vi "AO and DO Engine.vi"(0 "Unique Notifier Name":string="Not a Name", 11 "AO Channel":string[](array[string])) -> ()   [LabVIEW 2016]
uses:
  External Power Control Type Defs/External Power Notifier Type.ctl
  External Power Control Type Defs/External Power Actions.ctl
  <vilib>/DAQmx/write.llb/DAQmx Write (Digital Bool 1Line 1Point).vi
  <vilib>/DAQmx/write.llb/DAQmx Write (Analog DBL 1Chan 1Samp).vi
  <vilib>/DAQmx/create/channels.llb/DAQmx Create Channel (DO-Digital Output).vi
  <vilib>/DAQmx/miscellaneous.llb/DAQmx Fill In Error Info.vi
  <vilib>/DAQmx/create/channels.llb/DAQmx Create Channel (AO-Voltage-Basic).vi
panel:
  in  "Power (%)":dbl
  in  "Quit":bool
  in  "Line On Off":bool
  # "Array Elements must be:\n\n1) AO Channel (e.g. Dev1/ao3)\n2) DO Channel (e.g. Dev1/port0/line16)"
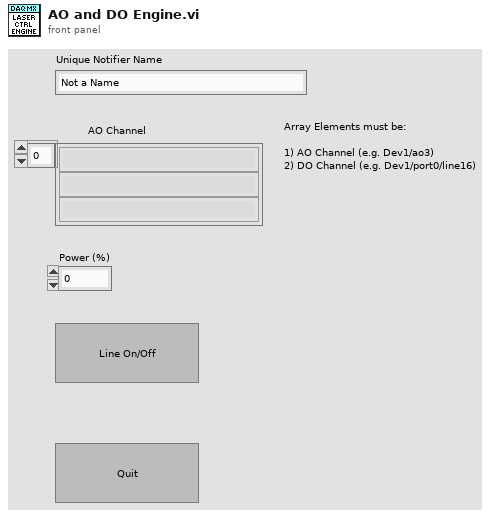
[diagram p1: front panel]
types:
  T1 = typedef "External Power Notifier Type.ctl" = cluster{"Actions":T2, "Wavelength":string, "Line On/Off":bool, "Power (%)":dbl, "Control Parameters":variant, "Cmd Done?":bool}
  T2 = typedef "External Power Actions.ctl" = enum16{"Line On/Off", "Set Power", "Set Ctrl Parameters", "Quit"}
  T3 = enum32{"Invalid", "Standard", "Closed", "Hidden", "Minimized", "Maximized"}
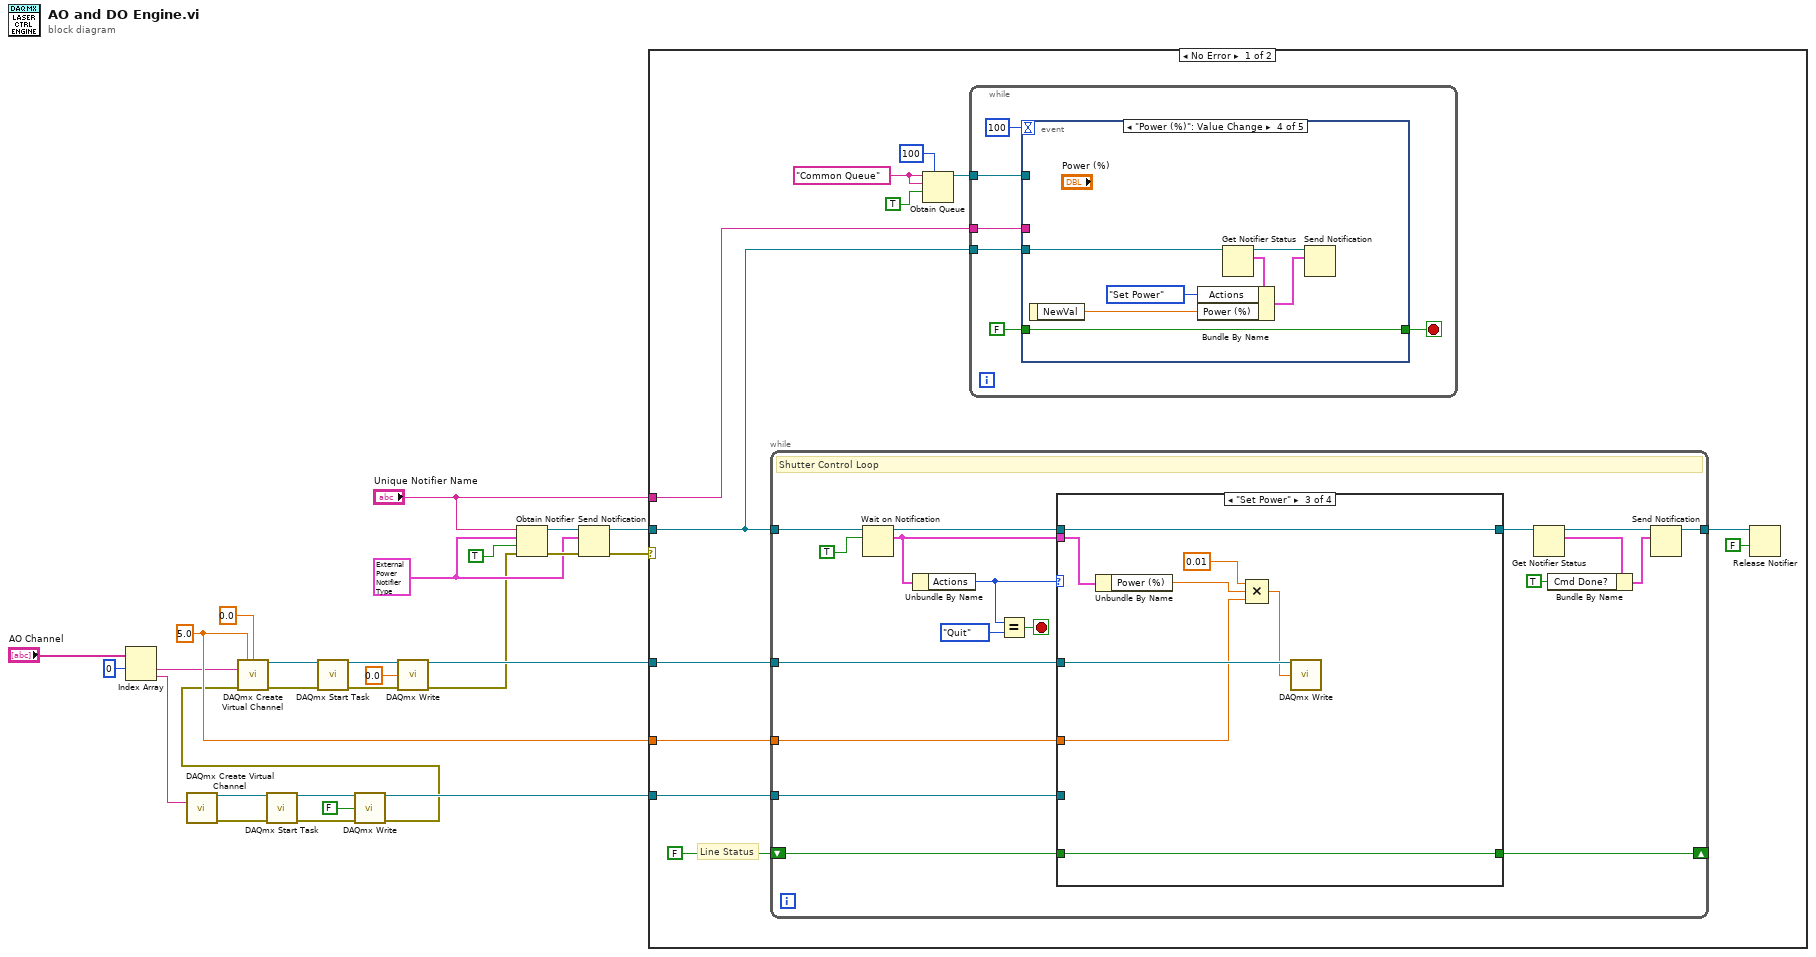
[diagram p0: block diagram]
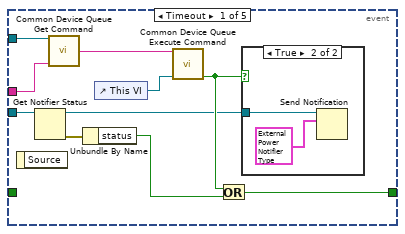
[diagram p2: hidden frame]
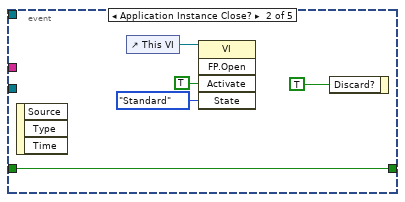
[diagram p4: hidden frame]
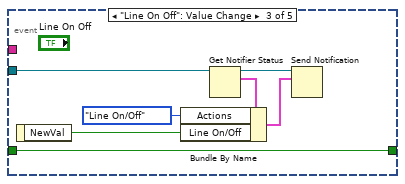
[diagram p5: hidden frame]
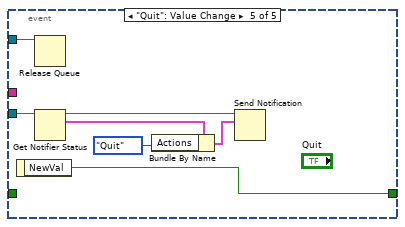
[diagram p6: hidden frame]
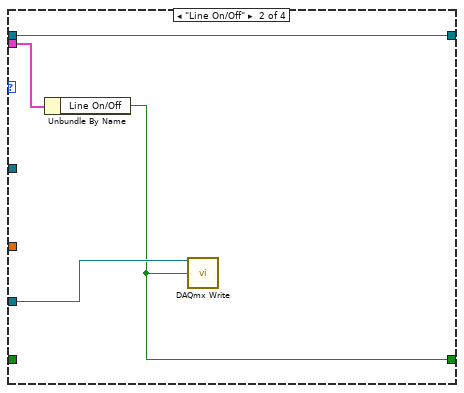
[diagram p8: hidden frame]
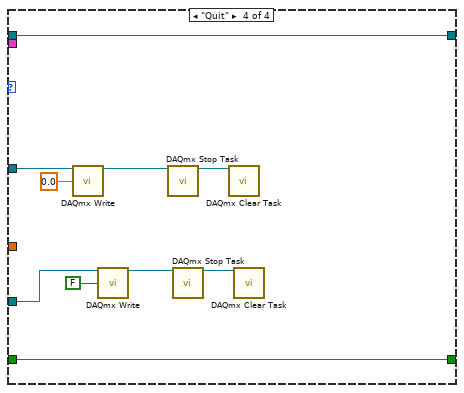
[diagram p9: hidden frame]
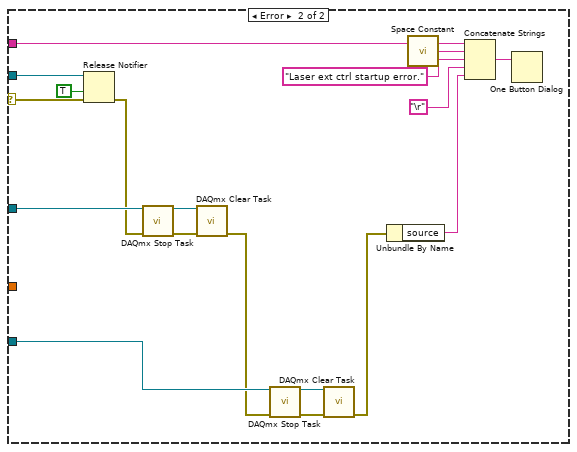
[diagram p10: hidden frame]
diagram:
  w18 = 5.0 ("maximum value")
  w23 = T1 {"Actions"=enum."Set Power", "Wavelength"="", "Line On/Off"=FALSE, "Power (%)"=0.0, "Control Parameters"=variant, "Cmd Done?"=FALSE} ("External Ctrl")
  n1 = Index Array(array="AO Channel", index #1=0 ("index")) -> (element #1=w9:string, element #2=w1:string)  [unwired: 1 in]
  n2 = call-poly <vilib>:"DAQmx Create Virtual Channel.vi"("lines"=w1) -> ("task out"=w7:refnum<k21>, "error out"=w8:errorcluster)  [unwired: 13 in]
  n3 = call <vilib>:"DAQmx Start Task.vi"("task/channels in"=w7, "error in"=w8) -> ("task out"=w6:refnum<k21>, "error out"=w4:errorcluster)  [unwired: 12 out]
  n4 = call-poly <vilib>:"DAQmx Write.vi"("task/channels in"=w6, "data"=FALSE, "error in"=w4) -> ("task out"=w3:refnum<k21>, "error out"=w2:errorcluster)  [unwired: 10 in, 1 out]
  n5 = call-poly <vilib>:"DAQmx Create Virtual Channel.vi"("maximum value"=w18, "minimum value"=0.0, "physical channels"=w9, "error in"=w2) -> ("task out"=w14:refnum<k21>, "error out"=w13:errorcluster)  [unwired: 10 in]
  n6 = call <vilib>:"DAQmx Start Task.vi"("task/channels in"=w14, "error in"=w13) -> ("task out"=w12:refnum<k21>, "error out"=w11:errorcluster)  [unwired: 12 out]
  n7 = call-poly <vilib>:"DAQmx Write.vi"("task/channels in"=w12, "data"=0.0, "error in"=w11) -> ("task out"=w16:refnum<k21>, "error out"=w10:errorcluster)  [unwired: 10 in, 1 out]
  n8 = Obtain Notifier(name (unnamed)="Unique Notifier Name", notification data type=w23, create if not found? (T)=TRUE, error in (no error)=w10) -> (notifier out=w26:refnum<notifier>, error out=w25:errorcluster)  [unwired: 1 out]
  n9 = Send Notification(notification=w23, notifier=w26, error in (no error)=w25) -> (notifier out=w24:refnum<notifier>, error out=w22:errorcluster)
  n10 = case shown="No Error" w22 {
    selector: w22 -> [_ w141]
    tunnel: w16 -> [w39 w132]
    tunnel: w24 -> [w37 w142]
    tunnel: "Unique Notifier Name" -> [w36 w140]
    tunnel: w18 -> [w30 _]
    tunnel: w3 -> [w28 w129]
    frame No Error {
      w35 = "Common Queue" ("Unique Notifier Name")
      # "Line Status"
      n11 = while {
        tunnel: w37 -> [w93]
        tunnel: w39 -> [w99]
        tunnel: [w94] -> w29
        shift-right: [w86] -> _
        shift-left: FALSE -> [w87]
        tunnel: w30 -> [w85]
        tunnel: w28 -> [w84]
        stop <- w100 stop-if-true
        # "Shutter Control Loop"
        n12 = Wait on Notification(notifier=w93, ignore previous (F)=TRUE) -> (notifier out=w92:refnum<notifier>, notification=w91:T1)  [unwired: 2 in, 2 out]
        n13 = Unbundle By Name(w91) -> ("Actions"=w90:T2)
        n14 = Equal?(x=w90, y=External_Power_Actions."Quit") -> (x = y?=w100:bool)
        n15 = case shown="\"Set Power\"" w90 {
          tunnel: w92 -> [w103 w107 w115 w125]
          tunnel: w99 -> [_ _ w110 w122]
          tunnel: [w103 w107 w115 w125] -> w97
          tunnel: w91 -> [_ w106 w114 _]
          tunnel: w87 -> [w102 _ w111 w124]
          tunnel: [w102 w104 w111 w124] -> w86
          tunnel: w85 -> [_ _ w108 _]
          tunnel: w84 -> [_ w105 _ w118]
          frame Default {
          }
          frame "Line On/Off" {
            n16 = Unbundle By Name(w106) -> ("Line On/Off"=w104:bool)
            n17 = call-poly <vilib>:"DAQmx Write.vi"("task/channels in"=w105, "data"=w104) -> ()  [unwired: 11 in, 3 out]
          }
          frame "Set Power" {
            n18 = Unbundle By Name(w114) -> ("Power (%)"=w113:dbl)
            n19 = Compound Arithmetic op=MULTIPLY(0.01 ("value"), w113, w108) -> (w109:dbl)
            n20 = call-poly <vilib>:"DAQmx Write.vi"("task/channels in"=w110, "data"=w109) -> ()  [unwired: 11 in, 3 out]
          }
          frame "Quit" {
            n21 = call-poly <vilib>:"DAQmx Write.vi"("task/channels in"=w122, "data"=0.0) -> ("task out"=w120:refnum<k21>)  [unwired: 11 in, 2 out]
            n22 = call-poly <vilib>:"DAQmx Write.vi"("task/channels in"=w118, "data"=FALSE) -> ("task out"=w116:refnum<k21>)  [unwired: 11 in, 2 out]
            n23 = call <vilib>:"DAQmx Stop Task.vi"("task/channels in"=w120) -> ("task out"=w121:refnum<k21>)  [unwired: 13 in, 1 out]
            n24 = call <vilib>:"DAQmx Stop Task.vi"("task/channels in"=w116) -> ("task out"=w117:refnum<k21>)  [unwired: 13 in, 1 out]
            n25 = call <vilib>:"DAQmx Clear Task.vi"("task in"=w121) -> ()  [unwired: 14 in, 1 out]
            n26 = call <vilib>:"DAQmx Clear Task.vi"("task in"=w117) -> ()  [unwired: 14 in, 1 out]
          }
        }
        n27 = Get Notifier Status(notifier=w97) -> (notifier out=w95:refnum<notifier>, current notification=w98:T1)  [unwired: 1 in, 3 out]
        n28 = Bundle By Name(cluster=w98, "Cmd Done?"=TRUE ("Received?")) -> (w88:T1)
        n29 = Send Notification(notification=w88, notifier=w95) -> (notifier out=w94:refnum<notifier>)  [unwired: 1 in, 1 out]
      }
      n30 = Obtain Queue(max queue size (-1, unlimited)=100, name (unnamed)=w35, element data type=w35, create if not found? (T)=TRUE) -> (queue out=w32:refnum<queue>)  [unwired: 1 in, 2 out]
      n31 = while {
        tunnel: w32 -> [w45]
        tunnel: w37 -> [w42]
        tunnel: w36 -> [w40]
        stop <- w41 stop-if-true
        n32 = event shown="[3] \"Power (%)\": Value Change" {
          selector: _ -> [_ _ _ _ _]
          dyn-events: _ -> [_ _ _ _ _]
          timeout: 100 -> [_ _ _ _ _]
          tunnel: w45 -> [w53 _ _ _ w78]
          tunnel: FALSE -> [_ w62 w65 w72 _]
          tunnel: w42 -> [w55 _ w69 w76 w79]
          tunnel: [w48 w62 w65 w72 w83] -> w41
          tunnel: w40 -> [w52 _ _ _ _]
          event Timeout {
            n33 = event-data() -> ()  [unwired: 1 in, 1 out]
            n34 = Get Notifier Status(notifier=w55) -> (notifier out=w46:refnum<notifier>, error out=w54:errorcluster)  [unwired: 1 in, 3 out]
            n35 = call "Common Device Queue Get Command.vi"("Common Queue"=w53, "Notifier Name"=w52) -> ("Command"=w51:string)  [unwired: 12 in, 1 out]
            n36 = Unbundle By Name(w54) -> ("status"=w49:bool)
            n37 = control-ref of="This VI"() -> (w50:refnum<vi>)
            n38 = call "Common Device Queue Execute Command.vi"("Common Command"=w51, "VI Refnum"=w50) -> ("Quit?"=w47:bool)  [unwired: 12 in, 1 out]
            n39 = Or(x=w47, y=w49) -> (x .or. y?=w48:bool)
            n40 = case shown="True" w47 {
              tunnel: w46 -> [_ w57]
              frame False {
              }
              frame True {
                n41 = Send Notification(notification=T1 {"Actions"=enum."Quit", "Wavelength"="", "Line On/Off"=FALSE, "Power (%)"=0.0, "Control Parameters"=variant, "Cmd Done?"=FALSE} ("External Ctrl"), notifier=w57) -> ()  [unwired: 1 in, 2 out]
              }
            }
          }
          event Application Instance Close? {
            n42 = event-data() -> ()  [unwired: 1 in, 3 out]
            n43 = control-ref of="This VI"() -> (w59:refnum<vi>)
            n44 = invoke class="VI" method="FP.Open"(reference=w59, "Activate"=TRUE ("Activate?"), "State"=T3."Standard") -> ()  [unwired: 2 in, 5 out]
            n45 = event-data("Discard?"=TRUE) -> ()  [unwired: 1 in, 1 out]
          }
          event "Line On Off": Value Change {
            n46 = event-data() -> ("NewVal"=w64:bool)  [unwired: 1 in]
            n47 = Get Notifier Status(notifier=w69) -> (notifier out=w68:refnum<notifier>, current notification=w67:T1)  [unwired: 1 in, 3 out]
            n48 = Bundle By Name(cluster=w67, "Actions"=External_Power_Actions."Line On/Off", "Line On/Off"=w64) -> (w66:T1)
            n49 = Send Notification(notification=w66, notifier=w68) -> ()  [unwired: 1 in, 2 out]
          }
          event "Power (%)": Value Change {
            n50 = event-data() -> ("NewVal"=w71:dbl)  [unwired: 1 in]
            n51 = Get Notifier Status(notifier=w76) -> (notifier out=w75:refnum<notifier>, current notification=w74:T1)  [unwired: 1 in, 3 out]
            n52 = Bundle By Name(cluster=w74, "Actions"=External_Power_Actions."Set Power", "Power (%)"=w71) -> (w73:T1)
            n53 = Send Notification(notification=w73, notifier=w75) -> ()  [unwired: 1 in, 2 out]
          }
          event "Quit": Value Change {
            n54 = event-data() -> ("NewVal"=w83:bool)  [unwired: 1 in]
            n55 = Release Queue(queue=w78) -> ()  [unwired: 2 in, 3 out]
            n56 = Get Notifier Status(notifier=w79) -> (notifier out=w82:refnum<notifier>, current notification=w81:T1)  [unwired: 1 in, 3 out]
            n57 = Bundle By Name(cluster=w81, "Actions"=External_Power_Actions."Quit") -> (w80:T1)
            n58 = Send Notification(notification=w80, notifier=w82) -> ()  [unwired: 1 in, 2 out]
          }
        }
      }
      n59 = Release Notifier(notifier=w29, force destroy? (F)=FALSE) -> ()  [unwired: 1 in, 3 out]
    }
    frame Error {
      n60 = Release Notifier(notifier=w142, force destroy? (F)=TRUE, error in (no error)=w141) -> (error out=w128:errorcluster)  [unwired: 2 out]
      n61 = call <vilib>:"DAQmx Stop Task.vi"("task/channels in"=w132, "error in"=w128) -> ("task out"=w134:refnum<k21>, "error out"=w133:errorcluster)  [unwired: 12 in]
      n62 = call <vilib>:"DAQmx Clear Task.vi"("task in"=w134, "error in"=w133) -> ("error out"=w127:errorcluster)  [unwired: 13 out]
      n63 = call <vilib>:"DAQmx Stop Task.vi"("task/channels in"=w129, "error in"=w127) -> ("task out"=w130:refnum<k21>, "error out"=w131:errorcluster)  [unwired: 12 in]
      n64 = call <vilib>:"DAQmx Clear Task.vi"("task in"=w130, "error in"=w131) -> ("error out"=w126:errorcluster)  [unwired: 13 out]
      n65 = Unbundle By Name(w126) -> ("source"=w135:string)
      n66 = call <vilib>:"Space Constant.vi"() -> ("String"=w138:string)
      n67 = Concatenate Strings(w140, w138, "Laser ext ctrl startup error." ("string"), "\r", w135) -> (w139:string)
      n68 = One Button Dialog(message=w139) -> ()  [unwired: 1 in, 1 out]
    }
  }
